vi "Destroy.vi"(8 "error in (no error)":errorcluster, 11 "BCReg":refnum<data-value>) -> (0 "error out":errorcluster)   [LabVIEW 2017, in "BusController.lvlib" / "BCReg.lvclass"]
uses:
  BCReg.lvclass
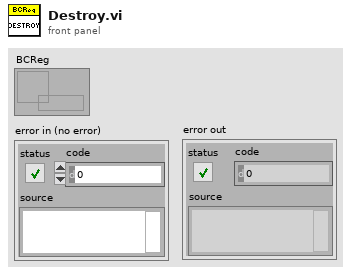
[diagram p1: front panel]
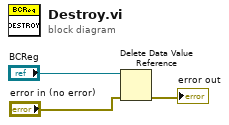
[diagram p0: block diagram]
diagram:
  n1 = Delete Data Value Reference(data value reference="BCReg", error in="error in (no error)") -> (error out=→"error out":errorcluster)  [unwired: 1 out]
